vi "Process.vi"(8 "error in (no error)":errorcluster, 9 "System Status Ref.":refnum<vi>, 10 "pound in":refnum<class "Pound.lvclass">, 11 "qbus in":refnum<class "Qbus.lvclass">) -> (0 "error out":errorcluster)   [LabVIEW 2015, in "CopyUtility.lvlib"]
doc: "Implements timer tasks that other processes register by sending Qbus messages to those processes."
uses:
  CopyUtility.lvlib
  <vilib>/addons/Qbus/Qbus.lvclass
  <vilib>/NI/Software Watchdog/Pound/Pound.lvclass
  controls/ProcessState.ctl
  <vilib>/addons/TimerProcess/controls/taskType.ctl
  <vilib>/NI/Software Watchdog/Watchdog/Watchdog.lvclass
  <vilib>/addons/TimerProcess/TimerProcess.lvlib
  FileHandler/FileHandler.lvlib
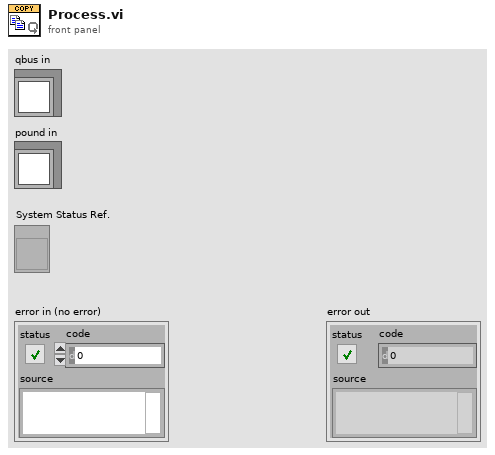
[diagram p1: front panel]
types:
  T1 = typedef "CopyUtility.lvlib/ProcessState.ctl" = cluster{"FileList":path[], "TimerTaskName":string, "Counts":u64}
  T2 = typedef "TimerProcess.lvlib/taskType.ctl" = enum16{"single", "repeat"}
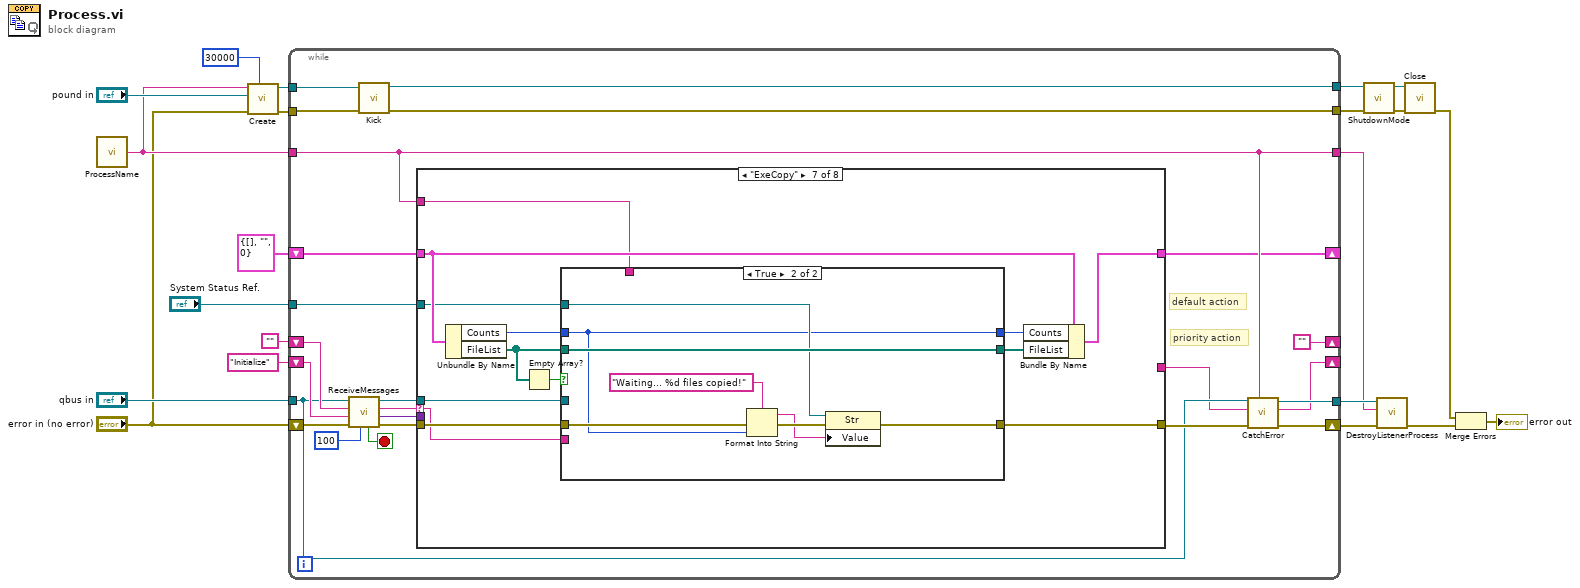
[diagram p0: block diagram]
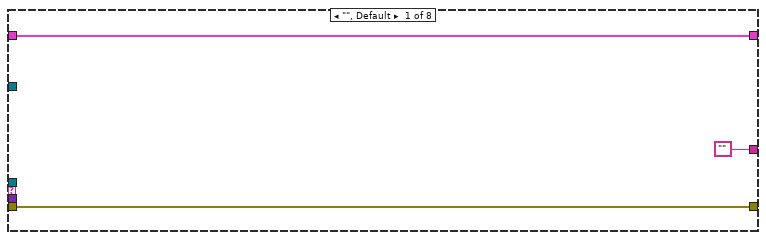
[diagram p2: hidden frame]
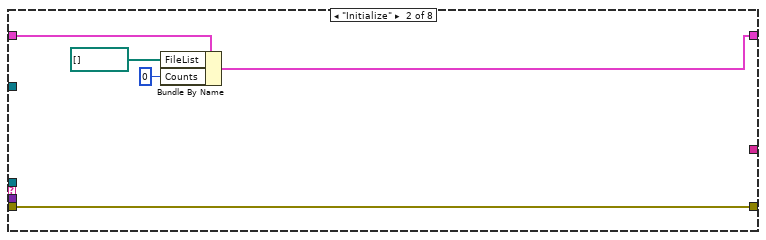
[diagram p3: hidden frame]
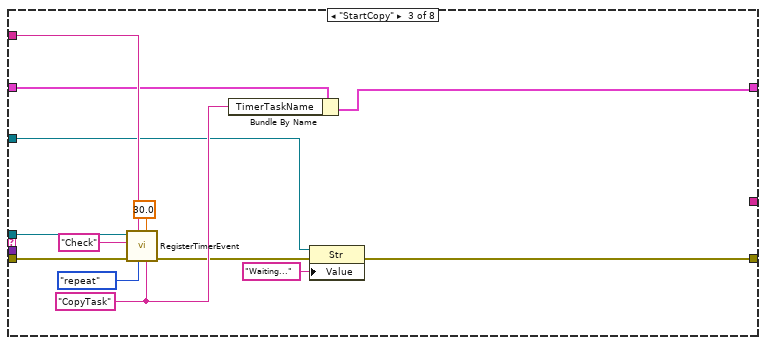
[diagram p4: hidden frame]
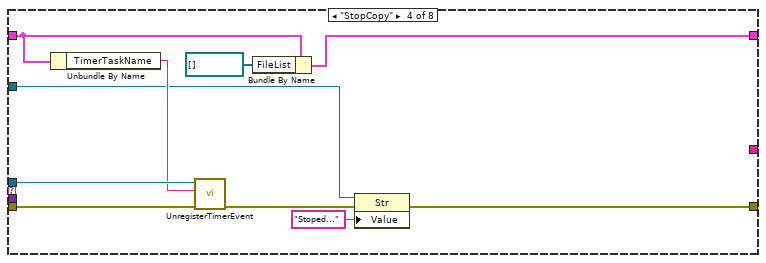
[diagram p5: hidden frame]
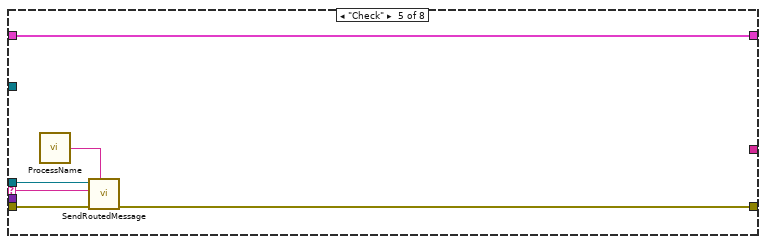
[diagram p6: hidden frame]
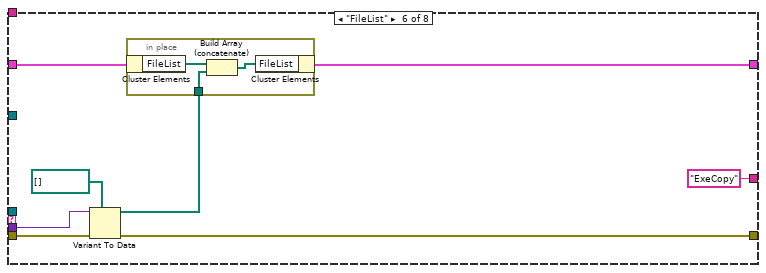
[diagram p7: hidden frame]
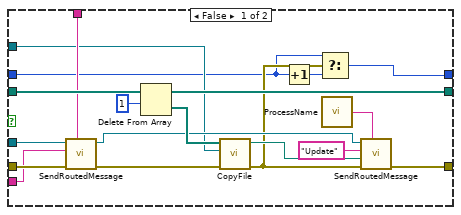
[diagram p8: hidden frame]
diagram:
  n1 = call "ProcessName.vi"() -> ("process name"=w12:string)  [unwired: 5 in]
  n2 = call <vilib>:"Create.vi"("Execution Timeout (ms)"=u32 30000, "error in (no error)"="error in (no error)", "Pound"="pound in", "Name"=w12) -> ("error out"=w14:errorcluster, "Watchdog"=w13:refnum<data-value>)  [unwired: 6 in]
  n3 = while {
    shift-right: [""] -> _
    shift-left: "" -> [w43]
    tunnel: "qbus in" -> [w27]
    tunnel: w12 -> [w34]
    tunnel: [w36] -> w19
    tunnel: [w34] -> w18
    shift-right: [w35] -> _
    shift-left: "Initialize" -> [w38]
    tunnel: w14 -> [w32]
    tunnel: w13 -> [w31]
    tunnel: [w30] -> w7
    tunnel: [w29] -> w8
    shift-right: [w37] -> w20
    shift-left: "error in (no error)" -> [w45]
    shift-right: [w24] -> _
    shift-left: T1 {"FileList"=[], "TimerTaskName"="", "Counts"=0} ("ProcessState") -> [w25]
    tunnel: "System Status Ref." -> [w22]
    stop <- w44 stop-if-true
    # "priority action"
    # "default action"
    n4 = call "ReceiveMessages.vi"("timeout(100)"=100, "error in (no error)"=w45, "priority action"=w38, "default action"=w43, "qbus in"=w27) -> ("error out"=w42:errorcluster, "message value"=w39:variant, "action"=w28:string, "qbus out"=w40:refnum<class "Qbus.lvclass">, "exit"=w44:bool)  [unwired: 2 in]
    n5 = call <vilib>:"Kick.vi"("error in (no error)"=w32, "Watchdog"=w31) -> ("error out"=w29:errorcluster, "Watchdog"=w30:refnum<data-value>)  [unwired: 8 in]
    n6 = case shown="\"ExeCopy\"" w28 {
      selector: w28 -> [_ _ _ _ w79 _ w98 _]
      tunnel: w42 -> [w48 w53 w63 w75 w82 w90 w103 w134]
      tunnel: w40 -> [_ _ w62 w76 w81 _ w99 _]
      tunnel: [w48 w53 w54 w68 w78 w87 w102 w134] -> w33
      tunnel: w39 -> [_ _ _ _ _ w89 _ _]
      tunnel: w34 -> [_ _ w61 _ _ _ w97 _]
      tunnel: w25 -> [w47 w52 w60 w73 w77 w85 w106 w135]
      tunnel: [w47 w51 w58 w71 w77 w83 w105 w135] -> w24
      tunnel: ["" _ _ _ _ "ExeCopy" _ _] -> w23
      tunnel: w22 -> [_ _ w56 w67 _ _ w96 _]
      frame "", Default {
      }
      frame "Initialize" {
        n7 = Bundle By Name(cluster=w52, "FileList"=path[] [], "Counts"=u64 0) -> (w51:T1)
      }
      frame "StartCopy" {
        w59 = "CopyTask" ("timer task name")
        n8 = call <vilib>:"RegisterTimerEvent.vi"("timer task name"=w59, "interval (sec)"=30.0, "type"=taskType."repeat", "process name"=w61, "error in (no error)"=w63, "callback action"="Check", "qbus in"=w62) -> ("error out"=w57:errorcluster)  [unwired: 3 in, 1 out]
        n9 = Bundle By Name(cluster=w60, "TimerTaskName"=w59) -> (w58:T1)
        n10 = property class="Str"(reference=w56, error in=w57, "Value"="Waiting...") -> (error out=w54:errorcluster)  [unwired: 1 out]
      }
      frame "StopCopy" {
        n11 = Unbundle By Name(w73) -> ("TimerTaskName"=w74:string)
        n12 = call <vilib>:"UnregisterTimerEvent.vi"("error in (no error)"=w75, "timer task name"=w74, "qbus in"=w76) -> ("error out"=w69:errorcluster)  [unwired: 7 in, 1 out]
        n13 = Bundle By Name(cluster=w73, "FileList"=path[] []) -> (w71:T1)
        n14 = property class="Str"(reference=w67, error in=w69, "Value"="Stoped...") -> (error out=w68:errorcluster)  [unwired: 1 out]
      }
      frame "Check" {
        n15 = call "ProcessName.vi"() -> ("process name"=w80:string)  [unwired: 5 in]
        n16 = call <vilib>:"SendRoutedMessage.vi"("listener process"=w80, "error in (no error)"=w82, "message name"=w79, "Qbus in"=w81) -> ("error in (no error)"=w78:errorcluster)  [unwired: 6 in, 1 out]
      }
      frame "FileList" {
        n17 = Variant To Data(error in=w90, type=path[] [], Variant=w89) -> (data=w84:path[], error out=w87:errorcluster)
        n18 = in-place {
          in-place-border: w84 -> [w92]
          n19 = in-place-cluster #1(w85) -> ("FileList"=w93:path[])
          n20 = Build Array (concatenate)(w93, w92) -> (w91:path[])
          n21 = in-place-cluster #1("FileList"=w91) -> (w83:T1)
        }
      }
      frame "ExeCopy" {
        n22 = Unbundle By Name(w106) -> ("Counts"=w95:u64, "FileList"=w100:path[])
        n23 = Empty Array?(array=w100) -> (empty?=w101:bool)
        n24 = case shown="True" w101 {
          tunnel: w100 -> [w125 w133]
          tunnel: [w123 w133] -> w104
          tunnel: w103 -> [w117 w130]
          tunnel: [w112 w132] -> w102
          tunnel: w99 -> [w118 _]
          tunnel: w98 -> [w116 _]
          tunnel: w97 -> [w115 _]
          tunnel: w96 -> [w111 w131]
          tunnel: w95 -> [w107 w127]
          tunnel: [w108 w127] -> w94
          frame False {
            n25 = call <vilib>:"SendRoutedMessage.vi"("listener process"=w115, "error in (no error)"=w117, "message name"=w116, "Qbus in"=w118) -> ("error in (no error)"=w114:errorcluster, "Qbus out"=w113:refnum<class "Qbus.lvclass">)  [unwired: 6 in]
            n26 = Delete From Array(array=w125, length=1) -> (deleted portion=w122:path[], array with subset deleted=w123:path[])  [unwired: 1 in]
            n27 = call "CopyFile.vi"("error in (no error)"=w114, "System Status Ref."=w111, "Source File"=w122) -> ("error out"=w110:errorcluster, "Source File dup."=w121:path)  [unwired: 7 in]
            n28 = Increment(x=w107) -> (x+1=w109:u64)
            n29 = Select(t=w107, s=w110, f=w109) -> (s? t:f=w108:u64)
            n30 = call "ProcessName.vi"() -> ("process name"=w119:string)  [unwired: 5 in]
            n31 = call <vilib>:"SendRoutedMessage.vi"("listener process"=w119, "error in (no error)"=w110, "message value"=w121, "message name"="Update", "Qbus in"=w113) -> ("error in (no error)"=w112:errorcluster)  [unwired: 5 in, 1 out]
          }
          frame True {
            n32 = Format Into String(format string="Waiting... %d files copied!" ("Value"), error in=w130, w127) -> (resulting string=w126:string, error out=w129:errorcluster)  [unwired: 1 in]
            n33 = property class="Str"(reference=w131, error in=w129, "Value"=w126) -> (error out=w132:errorcluster)  [unwired: 1 out]
          }
        }
        n34 = Bundle By Name(cluster=w106, "Counts"=w94, "FileList"=w104) -> (w105:T1)
      }
      frame "Exit" {
      }
    }
    n35 = call <vilib>:"CatchError.vi"("source"=w34, "error in (no error)"=w33, "next action in"=w23, "Qbus in"=w27) -> ("error out"=w37:errorcluster, "next action out"=w35:string, "Qbus out"=w36:refnum<class "Qbus.lvclass">)  [unwired: 5 in]
  }
  n36 = call <vilib>:"ShutdownMode.vi"("error in (no error)"=w8, "Watchdog"=w7) -> ("error out"=w9:errorcluster, "Watchdog"=w10:refnum<data-value>)  [unwired: 8 in]
  n37 = call <vilib>:"DestroyListenerProcess.vi"("error in (no error)"=w20, "process name"=w18, "Qbus in"=w19) -> ("error in (no error)"=w5:errorcluster)  [unwired: 7 in, 1 out]
  n38 = call <vilib>:"Close.vi"("error in (no error)"=w9, "Watchdog"=w10) -> ("error out"=w6:errorcluster)  [unwired: 9 in]
  n39 = Merge Errors(w6, w5) -> (→"error out":errorcluster)
